vi "Get All Paths Calibration.vi"(8 "Error In":errorcluster) -> (0 "Error Out":errorcluster, 3 "All Paths":T1(array[cluster]))   [LabVIEW 2020, in "PathControl.lvclass"]
doc: "Gets all already calibrated paths.\nThis should only be used by the calibration UI in the Path Control class"
uses:
  PathControl.lvclass
  Measurements Specific Paths.ctl
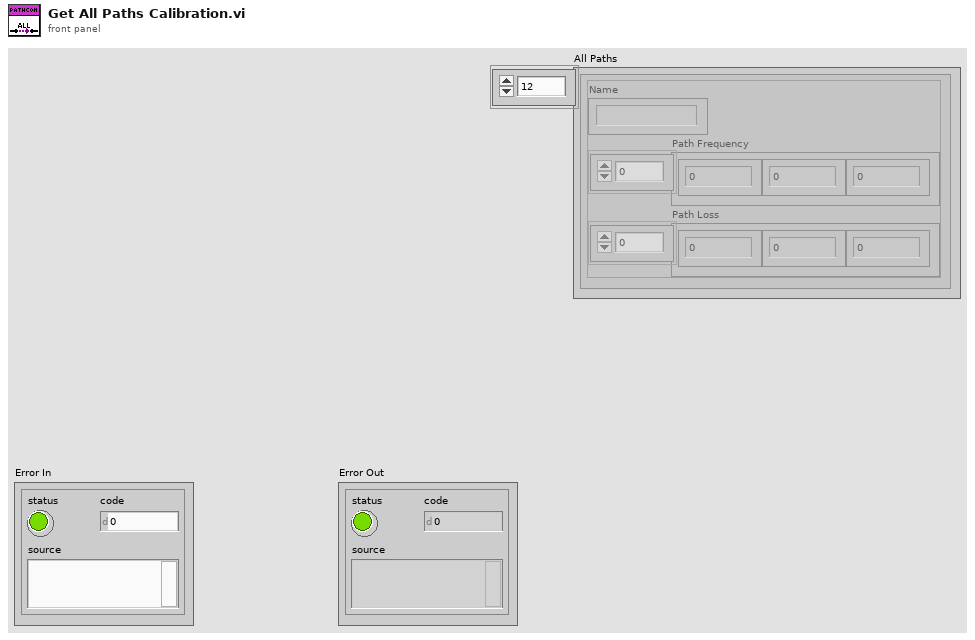
[diagram p1: front panel]
types:
  T1 = cluster{"Name":string, "Path Frequency":dbl[], "Path Loss":dbl[]}[]
  T2 = typedef "PathControl.lvclass/Measurements Specific Paths.ctl" = enum16{"No calibration", "Harmonics", "IMD", "S Parameter", "AM-AM", "MCCW-ACLR", "DC", "LCR", "Power Meter GUI", "RF Power"}
  T3 = cluster{"Name":string, "Path Frequency":dbl[], "Path Loss":dbl[]}
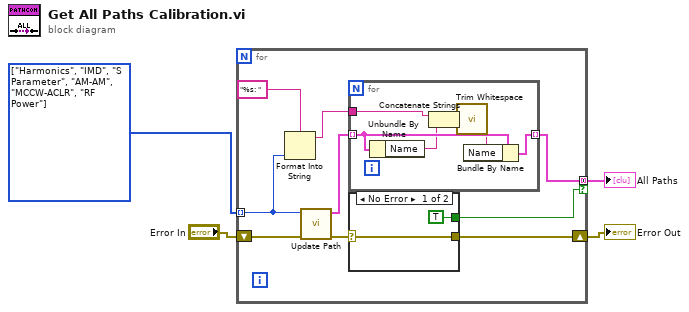
[diagram p0: block diagram]
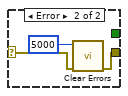
[diagram p2: hidden frame]
diagram:
  w3 = T2[] [enum."Harmonics", enum."IMD", enum."S Parameter", enum."AM-AM", enum."MCCW-ACLR", enum."RF Power"] items=["No calibration", "Harmonics", "IMD", "S Parameter", "AM-AM", "MCCW-ACLR", "DC", "LCR", "Power Meter GUI", "RF Power"]
  n1 = for {
    tunnel: w3 -> [w7] mode=indexing
    tunnel: [w5] -> w1 mode=concatenating if=w11
    shift-right: [w10] -> w2
    shift-left: "Error In" -> [w13]
    n2 = Format Into String(format string="%s: ", w7) -> (resulting string=w6:string)  [unwired: 2 in, 1 out]
    n3 = call "Update Path.vi"("Error In"=w13, "Measurement specfic paths"=w7) -> ("Error Out"=w12:errorcluster, "Current Paths"=w9:T1)  [unwired: 8 in]
    n4 = for {
      tunnel: w9 -> [w19] mode=indexing
      tunnel: w6 -> [w16]
      tunnel: [w18] -> w5 mode=indexing
      n5 = Unbundle By Name(w19) -> ("Name"=w17:string)
      n6 = Concatenate Strings(w16, w17) -> (w15:string)
      n7 = call <vilib>:"Trim Whitespace.vi"("string"=w15) -> ("trimmed string"=w14:string)  [unwired: 1 in]
      n8 = Bundle By Name(cluster=w19, "Name"=w14) -> (w18:T3)
    }
    n9 = case shown="No Error" w12 {
      selector: w12 -> [w20 w24]
      tunnel: [TRUE _] -> w11
      tunnel: [w20 w22] -> w10
      frame No Error {
      }
      frame Error {
        n10 = call <vilib>:"Clear Errors.vi"("error in (no error)"=w24, "specific error code to clear (0: all)"=5000) -> ("error out"=w22:errorcluster)  [unwired: 4 in, 1 out]
      }
    }
  }
  "Error Out" <- w2
  "All Paths" <- w1
